vi "Create Meas Plugin APIs - Multiple Converter.vi"(0 "logic vi in":refnum<vi>, 11 "error in":errorcluster) -> (4 "logic vi out":refnum<vi>, 6 "sub vi refrences":refnum<vi>[](array[refnum]), 15 "error out":errorcluster)   [LabVIEW 2021, in "Converter.lvlib"]
uses:
  Converter.lvlib
  <vilib>/Utility/miscctls.llb/LVPointTypeDef.ctl
  Path Functions/Path Functions.lvlib
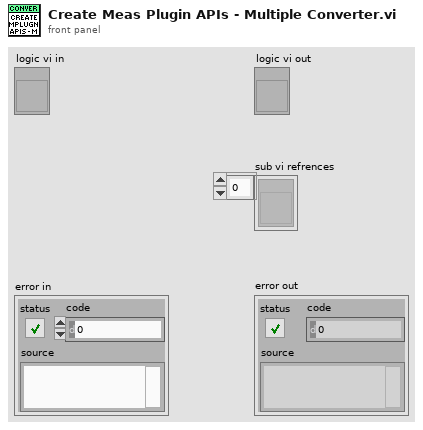
[diagram p1: front panel]
types:
  T1 = typedef "LVPointTypeDef.ctl" = cluster{"Horizontal":i16, "Vertical":i16}
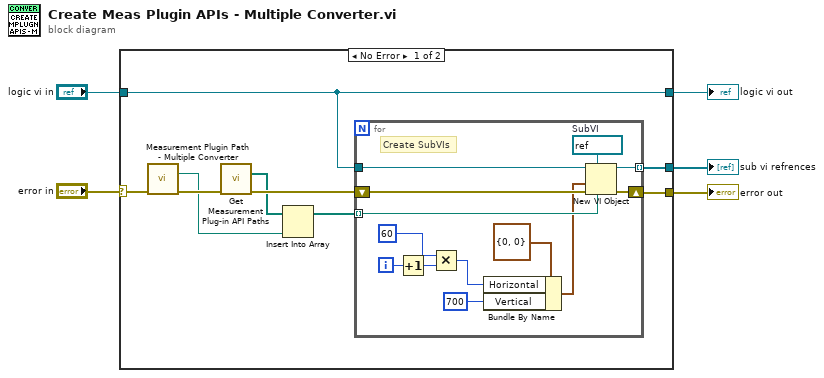
[diagram p0: block diagram]
diagram:
  n1 = case shown="No Error" "error in" {
    selector: "error in" -> [w8 w28]
    tunnel: [w12 _] -> w5
    tunnel: [w10 w28] -> w4
    tunnel: "logic vi in" -> [w9 w29]
    tunnel: [w9 w29] -> w1
    frame No Error {
      n2 = call "Measurement Plugin Path - Multiple Converter.vi"("error in"=w8) -> ("wrapper path"=w6:path, "error out"=w7:errorcluster)  [unwired: 2 in, 11 out]
      n3 = call "Get Measurement Plug-in API Paths.vi"("error in"=w7) -> ("meas plugin api paths"=w13:path[], "error out"=w14:errorcluster)  [unwired: 13 in]
      n4 = Insert Into Array(array=w13, new element=w6) -> (w11:path[])  [unwired: 1 in]
      n5 = for {
        tunnel: w11 -> [w26] mode=indexing
        tunnel: w9 -> [w25]
        tunnel: [w20] -> w12 mode=indexing
        shift-right: [w21] -> w10
        shift-left: w14 -> [w27]
        i -> [w18]
        w24 = refnum<vi> refnum  # SubVI
        # "Create SubVIs"
        n6 = Increment(x=w18) -> (x+1=w16:i32)
        n7 = Multiply(x=60 ("Vertical"), y=w16) -> (x*y=w15:i32)
        n8 = Bundle By Name(cluster=T1 {"Horizontal"=0, "Vertical"=0} ("location"), "Horizontal"=w15, "Vertical"=i16 700) -> (w22:T1)
        n9 = New VI Object(vi object class=w24, owner refnum=w25, position/next to=w22, 6:w26, 8:w27) -> (object refnum=w20:refnum<vi>, 0:w21:errorcluster)  [unwired: 3 in]
      }
    }
    frame Error {
    }
  }
  "sub vi refrences" <- w5
  "error out" <- w4
  "logic vi out" <- w1
